vi "TestRFGVRoom.vi"() -> (0 "error out":errorcluster, 2 "Pass":bool)   [LabVIEW 2015]
uses:
  LVClasses/Flags/ColorFlags.ctl
  TypeDef/RoomsActionEnum.ctl
  LVClasses/Room/Room.lvclass/Room.ctl
  LVClasses/Room/Read Flags.lvclass.vi
  LVClasses/Flags/Flags.lvclass
  LVClasses/Room/Room.lvclass
panel:
  out "Read Room 2":string
  out "Read Room 1":string
  out "Read Room 2":T1={"Flag State"=[1, 3, 5, 7]}
  out "Read Flag":string
  out "Write Flag":string
  in  "State":bool[](array[boolean])=[FALSE, FALSE, FALSE, FALSE]
  out "Flags Read 1":T1={"Flag State"=[1, 3, 5, 7]}
  out "Flags Write":T1={"Flag State"=[1, 3, 5, 7]}
  out "Flags Read 2":T1={"Flag State"=[1, 3, 5, 7]}
  in  "FGV Room":i32=102
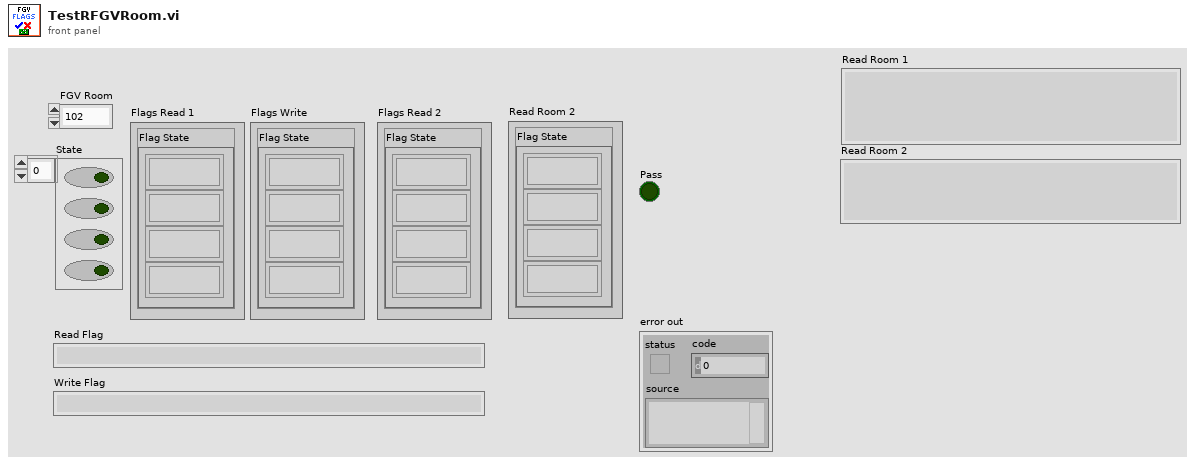
[diagram p1: front panel]
types:
  T1 = typedef "Flags.lvclass/ColorFlags.ctl" = cluster{"Flag State":u8[]}
  T2 = typedef "RoomsActionEnum.ctl" = enum16{"Init", "Add Room", "Remove Room", "Read Room", "Read Flag", "Read Flag State", "Write Flag State", "Read Flag Color", "Write Flag Color", "Read Bed Vacant", "Write Bed Vacant", "Read Personnel", "Add Personnel", "Remove Personnel", "Read Requests", "Add Request", "Remove Request", "Read Beacon ID", "Write Beacon ID", "Write Bed URL", "Read Bed URL", "Read Rooms Numbers", "Write Flag"}
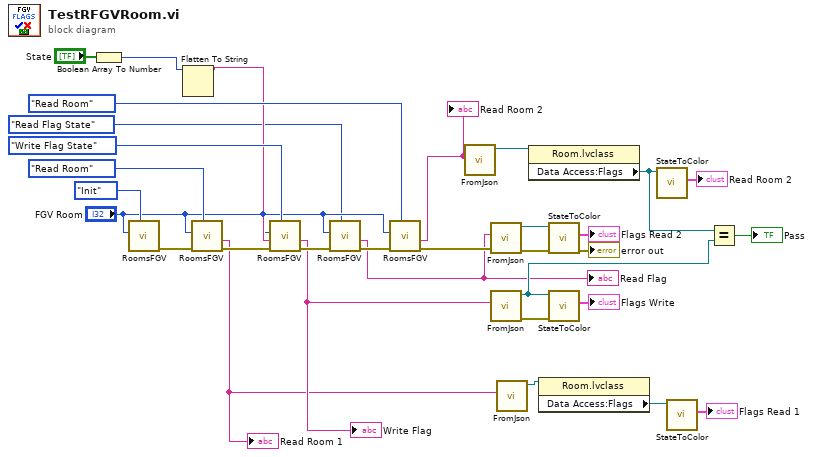
[diagram p0: block diagram]
diagram:
  n1 = Boolean Array To Number(Boolean array="State") -> (number=w13:u32)
  n2 = call "RoomsFGV.vi"("Actions"=RoomsActionEnum."Init", "Room"="FGV Room") -> ("error out"=w31:errorcluster)  [unwired: 8 in, 1 out]
  n3 = Flatten To String(anything=w13) -> (data string=w14:string)  [unwired: 3 in, 2 out]
  n4 = call "RoomsFGV.vi"("Actions"=RoomsActionEnum."Read Room", "error in (no error)"=w31, "Room"="FGV Room") -> ("error out"=w30:errorcluster, "Data Out"=w7:string)  [unwired: 7 in]
  "Read Room 1" <- w7
  n5 = call "RoomsFGV.vi"("Actions"=RoomsActionEnum."Write Flag State", "error in (no error)"=w30, "Data In"=w14, "Room"="FGV Room") -> ("error out"=w29:errorcluster, "Data Out"=w20:string)  [unwired: 6 in]
  "Write Flag" <- w20
  n6 = call "RoomsFGV.vi"("Actions"=RoomsActionEnum."Read Flag State", "error in (no error)"=w29, "Room"="FGV Room") -> ("error out"=w12:errorcluster, "Data Out"=w2:string)  [unwired: 7 in]
  "Read Flag" <- w2
  n7 = call "RoomsFGV.vi"("Actions"=RoomsActionEnum."Read Room", "error in (no error)"=w12, "Room"="FGV Room") -> ("error out"=w26:errorcluster, "Data Out"=w8:string)  [unwired: 7 in]
  "Read Room 2" <- w8
  n8 = call "FromJson.vi"("String"=w8) -> ("Room out"=w3:refnum<class "Room.lvclass">)  [unwired: 9 in, 1 out]
  n9 = call "FromJson.vi"("error in (no error)"=w26, "String"=w2) -> ("error out"=w25:errorcluster, "Flags out"=w9:refnum<class "Flags.lvclass">)  [unwired: 8 in]
  n10 = call "FromJson.vi"("String"=w20) -> ("error out"=w22:errorcluster, "Flags out"=w19:refnum<class "Flags.lvclass">)  [unwired: 9 in]
  n11 = call "FromJson.vi"("String"=w7) -> ("Room out"=w6:refnum<class "Room.lvclass">)  [unwired: 9 in, 1 out]
  n12 = property class="Room.lvclass"(reference=w3) -> ("Data Access:Flags"=w1:refnum<class "Flags.lvclass">)  [unwired: 1 in, 2 out]
  n13 = property class="Room.lvclass"(reference=w6) -> ("Data Access:Flags"=w5:refnum<class "Flags.lvclass">)  [unwired: 1 in, 2 out]
  n14 = call "StateToColor.vi"("error in (no error)"=w25, "Flags in"=w9) -> ("error out"=→"error out":errorcluster, "RoomNumFlags"=→"Flags Read 2":T1)  [unwired: 7 in, 1 out]
  n15 = call "StateToColor.vi"("error in (no error)"=w22, "Flags in"=w19) -> ("RoomNumFlags"=→"Flags Write":T1)  [unwired: 7 in, 2 out]
  n16 = call "StateToColor.vi"("Flags in"=w1) -> ("RoomNumFlags"=→"Read Room 2":T1)  [unwired: 8 in, 2 out]
  n17 = call "StateToColor.vi"("Flags in"=w5) -> ("RoomNumFlags"=→"Flags Read 1":T1)  [unwired: 8 in, 2 out]
  n18 = Equal?(x=w1, y=w19) -> (x = y?=→"Pass":bool)
